vi "Write Message Screen.vi"(8 "error in (no error)":errorcluster, 10 "Current Transaction":string, 11 "Simulated Display Console Actor in":refnum<class "Simulated Display Console Actor.lvclass">) -> (0 "error out":errorcluster, 3 "Simulated Display Console Actor out":refnum<class "Simulated Display Console Actor.lvclass">)   [LabVIEW 2019, in "Simulated Display Console Actor.lvlib" / "Simulated Display Console Actor.lvclass"]
uses:
  Simulated Display Console Actor.lvclass
  Simulated Display Console Actor.lvclass/Simulated Display Console Actor.ctl
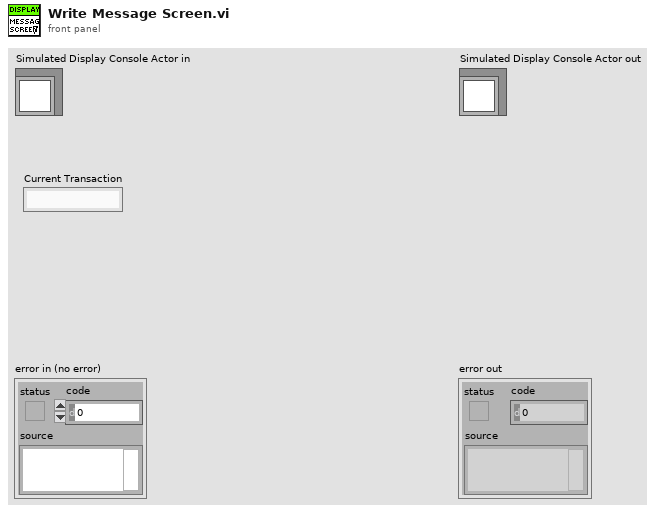
[diagram p1: front panel]
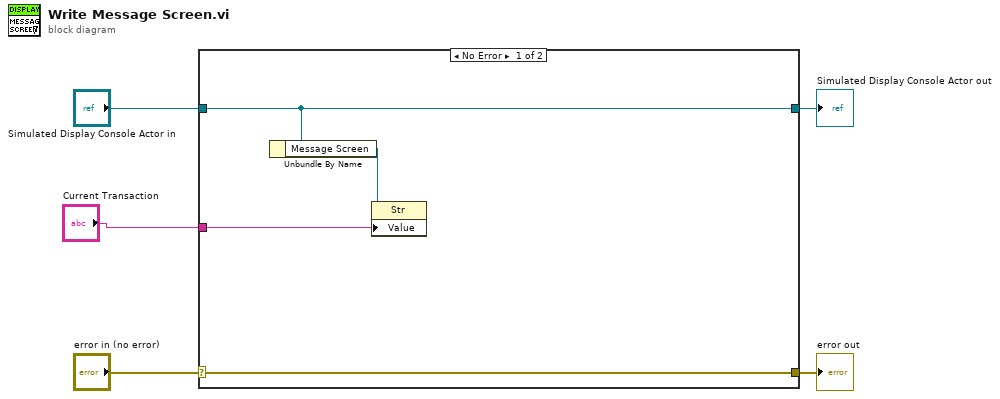
[diagram p0: block diagram]
diagram:
  n1 = case shown="No Error" "error in (no error)" {
    selector: "error in (no error)" -> [w9 w11]
    tunnel: [w9 w11] -> w4
    tunnel: [w8 w10] -> w2
    tunnel: "Simulated Display Console Actor in" -> [w8 w10]
    tunnel: "Current Transaction" -> [w6 _]
    frame No Error {
      n2 = Unbundle By Name(w8) -> ("Message Screen"=w7:refnum<vi>)
      n3 = property class="Str"(reference=w7, "Value"=w6) -> ()  [unwired: 1 in, 2 out]
    }
    frame Error {
    }
  }
  "error out" <- w4
  "Simulated Display Console Actor out" <- w2
